vi "Open Help Document.vi"(8 "error in (no error)":errorcluster, 11 "EPU452 in":refnum<class "EPU452.lvclass">) -> (0 "error out":errorcluster, 3 "EPU452 out":refnum<class "EPU452.lvclass">)   [LabVIEW 2018, in "EPU452.lvclass"]
uses:
  EPU452.lvclass
  <vilib>/Platform/browser.llb/Open URL in Default Browser (string).vi
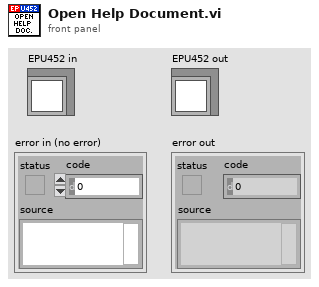
[diagram p1: front panel]
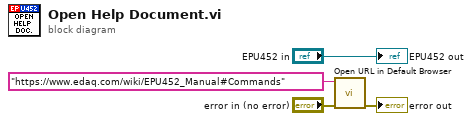
[diagram p0: block diagram]
diagram:
  n1 = call-poly <vilib>:"Open URL in Default Browser.vi"("error in (no error)"="error in (no error)", "URL"="https://www.edaq.com/wiki/EPU452_Manual#Commands") -> ("error out"=→"error out":errorcluster)  [unwired: 4 in, 1 out]
  "EPU452 out" <- "EPU452 in"
